vi "create-child-text.vi"(10 "results.text":string, 11 "results.data":string) -> (3 "Array":string[](array[string]))   [LabVIEW 2015]
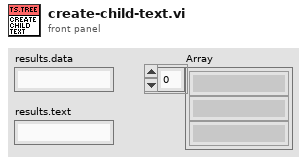
[diagram p1: front panel]
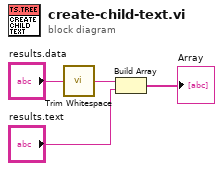
[diagram p0: block diagram]
diagram:
  n1 = call <vilib>:"Trim Whitespace.vi"("string"="results.data") -> ("trimmed string"=w1:string)  [unwired: 1 in]
  n2 = Build Array(w1, "results.text") -> (→"Array":string[])
